vi "LVClasse_SurfaceFloatWithPupil Write SurfaceFloatWithPupil.vi"(8 "error in (no error)":errorcluster, 10 "SurfaceFloatWithPupil":T1, 11 "SurfaceFloatWithPupil in":refnum<class "SurfaceFloatWithPupil.lvclass">) -> (0 "error out":errorcluster, 3 "SurfaceFloatWithPupil out":refnum<class "SurfaceFloatWithPupil.lvclass">)   [LabVIEW 2020, in "SurfaceFloatWithPupil.lvclass"]
uses:
  SurfaceFloatWithPupil.lvclass
  ClassID.ctl
  Handle creation.ctl
  SurfaceFloatWithPupil.lvclass/SurfaceFloatWithPupil.ctl
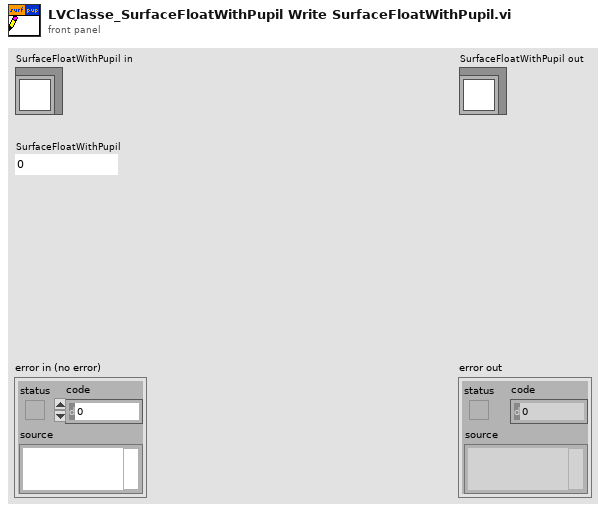
[diagram p1: front panel]
types:
  T1 = typedef "ClassID.ctl" = i64
  T2 = typedef "Handle creation.ctl" = enum16{"By ctor", "By write function"}
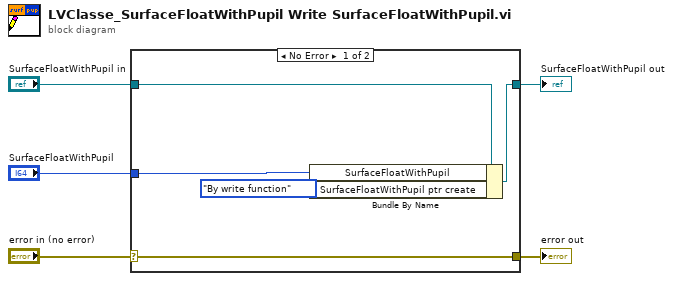
[diagram p0: block diagram]
diagram:
  n1 = case shown="No Error" "error in (no error)" {
    selector: "error in (no error)" -> [w10 w11]
    tunnel: [w10 w11] -> w4
    tunnel: [w8 w12] -> w2
    tunnel: "SurfaceFloatWithPupil in" -> [w9 w12]
    tunnel: "SurfaceFloatWithPupil" -> [w7 _]
    frame No Error {
      n2 = Bundle By Name(cluster=w9, "SurfaceFloatWithPupil"=w7, "SurfaceFloatWithPupil ptr create"=Handle_creation."By write function") -> (w8:refnum<class "SurfaceFloatWithPupil.lvclass">)
    }
    frame Error {
    }
  }
  "error out" <- w4
  "SurfaceFloatWithPupil out" <- w2
